vi "FMDLConfigKeithley6514AmmeterMode.vi"(8 "error in (no error)":errorcluster, 11 "VISA resource name":refnum<visa-resource-name>) -> (0 "error out":errorcluster, 3 "VISA resource name out":refnum<visa-resource-name>)   [LabVIEW 2018]
uses:
  <instrlib>/Keithley 6517/Keithley 6517.lvlib
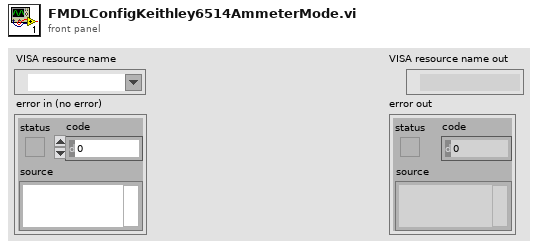
[diagram p1: front panel]
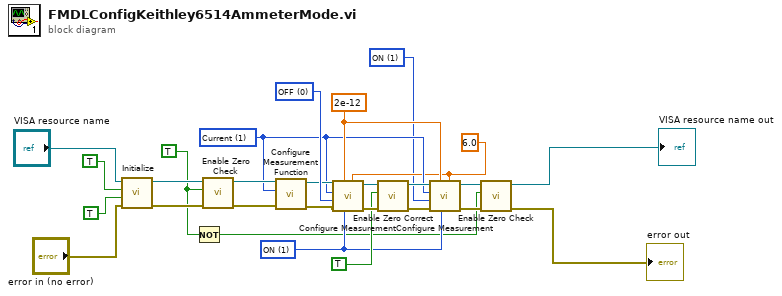
[diagram p0: block diagram]
diagram:
  w12 = 6.0 ("Display Resolution (6)")
  w1 = 1 items=["OFF", "ON", "ONCE"] ("Auto Range (1: ON)")
  w15 = 2e-12 ("Auto Range Value (2.0000000E+2)")
  w13 = 1 items=["OFF", "ON", "ONCE"] ("Auto Resolution (1: ON)")
  w23 = 0 items=["OFF", "ON", "ONCE"] ("Auto Range (1: ON)")
  w14 = 1 items=["Voltage", "Current", "Resistance", "Charge"] ("Measurement Function (0: Voltage)")
  w9 = TRUE ("Enable Zero Check (T: Enable)")
  n1 = call <instrlib>:"Initialize.vi"("error in (no error)"="error in (no error)", "Reset (True)"=TRUE, "ID Query (True)"=TRUE, "VISA resource name"="VISA resource name") -> ("error out"=w27:errorcluster, "VISA resource name out"=w26:refnum<visa-resource-name>)  [unwired: 6 in]
  n2 = Not(x=w9) -> (.not. x?=w8:bool)
  n3 = call <instrlib>:"Enable Zero Check.vi"("error in (no error)"=w27, "Enable Zero Check (T: Enable)"=w9, "VISA resource name"=w26) -> ("error out"=w25:errorcluster, "VISA resource name out"=w24:refnum<visa-resource-name>)  [unwired: 7 in]
  n4 = call <instrlib>:"Configure Measurement Function.vi"("error in (no error)"=w25, "Measurement Function (0: Voltage)"=w14, "VISA resource name"=w24) -> ("error out"=w21:errorcluster, "VISA resource name out"=w22:refnum<visa-resource-name>)  [unwired: 7 in]
  n5 = call <instrlib>:"Configure Measurement.vi"("Display Resolution (6)"=w12, "Auto Resolution (1: ON)"=w13, "Auto Range Value (2.0000000E+2)"=w15, "error in (no error)"=w21, "Auto Range (1: ON)"=w23, "Measurement Function (0: Voltage)"=w14, "VISA resource name"=w22) -> ("error out"=w20:errorcluster, "VISA resource name out"=w19:refnum<visa-resource-name>)  [unwired: 3 in]
  n6 = call <instrlib>:"Enable Zero Correct.vi"("error in (no error)"=w20, "Enable Zero Correct (F: Disable)"=TRUE, "VISA resource name"=w19) -> ("error out"=w16:errorcluster, "VISA resource name out"=w17:refnum<visa-resource-name>)  [unwired: 7 in]
  n7 = call <instrlib>:"Configure Measurement.vi"("Display Resolution (6)"=w12, "Auto Resolution (1: ON)"=w13, "Auto Range Value (2.0000000E+2)"=w15, "error in (no error)"=w16, "Auto Range (1: ON)"=w1, "Measurement Function (0: Voltage)"=w14, "VISA resource name"=w17) -> ("error out"=w10:errorcluster, "VISA resource name out"=w11:refnum<visa-resource-name>)  [unwired: 3 in]
  n8 = call <instrlib>:"Enable Zero Check.vi"("error in (no error)"=w10, "Enable Zero Check (T: Enable)"=w8, "VISA resource name"=w11) -> ("error out"=→"error out":errorcluster, "VISA resource name out"=→"VISA resource name out":refnum<visa-resource-name>)  [unwired: 7 in]
